vi "interp type 2.vi"(1 "NaN":dbl[][](array[numeric]) format="%.2f", 2 "Remove front and end":bool) -> (0 "Interpolated":dbl[][](array[numeric]) format="%.2f")   [LabVIEW 2016]
uses:
  <vilib>/Analysis/1siggen.llb/Ramp Pattern by Samples.vi
  <vilib>/Analysis/NI_AALBase.lvlib
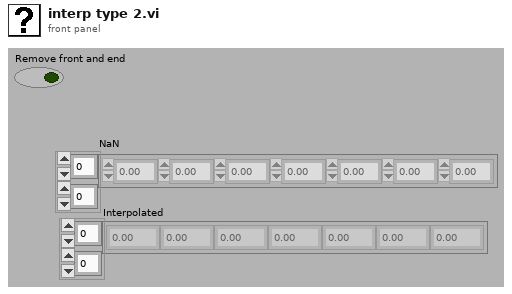
[diagram p1: front panel]
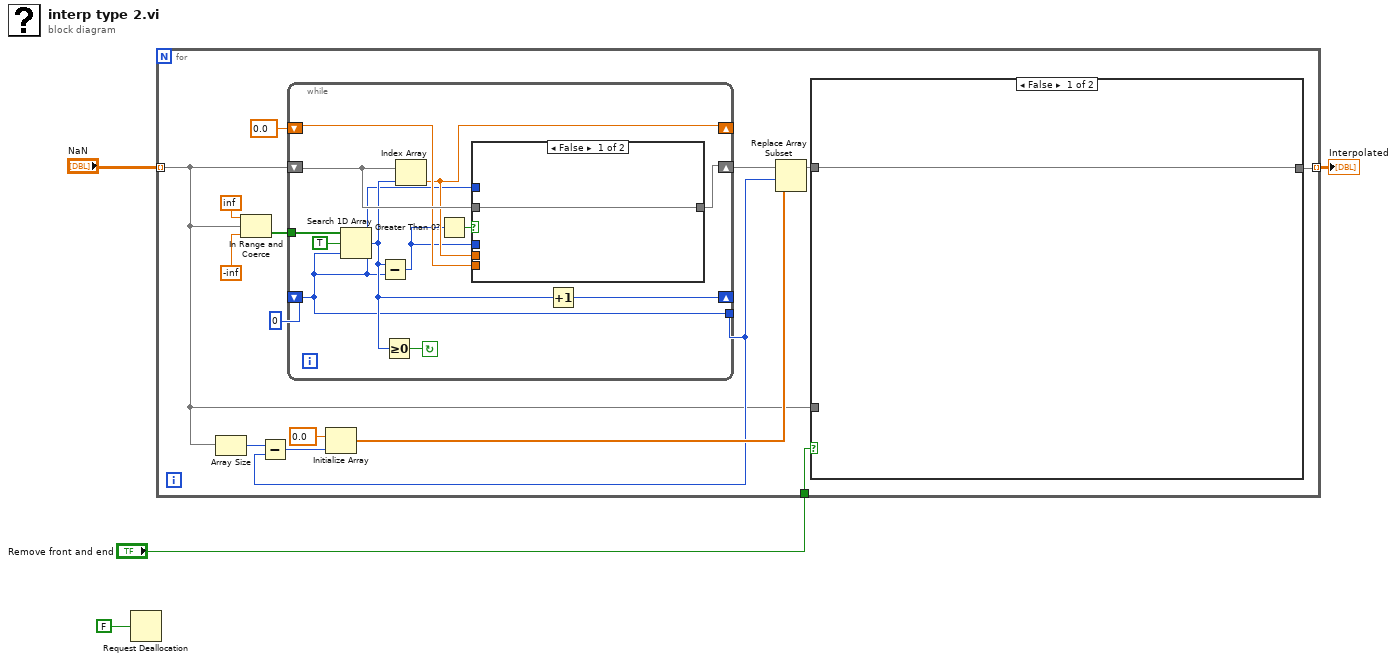
[diagram p0: block diagram]
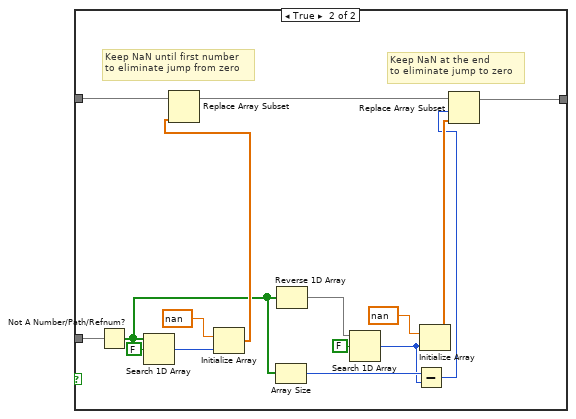
[diagram p2: hidden frame]
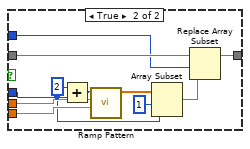
[diagram p3: hidden frame]
diagram:
  n1 = Request Deallocation(FALSE ("flag")) -> ()
  n2 = for {
    tunnel: "NaN" -> [w8] mode=indexing
    tunnel: [w6] -> w3 mode=indexing
    tunnel: "Remove front and end" -> [w5]
    n3 = Array Size(array=w8) -> (size(s)=w14:i32)
    n4 = In Range and Coerce(upper limit=inf, x=w8, lower limit=-inf) -> (In Range?=w17:bool[])  [unwired: 1 out]
    n5 = while {
      tunnel: w17 -> [w48]
      shift-right: [w38] -> _
      shift-left: 0 -> [w37]
      shift-right: [w43] -> w11
      shift-left: w8 -> [w46]
      shift-right: [w44] -> _
      shift-left: 0.0 ("Numeric") -> [w45]
      tunnel: [w37] -> w9
      stop <- w41 continue-if-true
      n6 = Search 1D Array(1D array=w48, element=TRUE, start index (0)=w37) -> (index of element=w42:i32)
      n7 = Subtract(x=w42, y=w37) -> (x-y=w39:i32)
      n8 = Greater Or Equal To 0?(x=w42) -> (x >= 0?=w41:bool)
      n9 = Index Array(array=w46, index=w42) -> (element=w44:dbl)
      n10 = Greater Than 0?(x=w39) -> (x > 0?=w40:bool)
      n11 = case shown="False" w40 {
        tunnel: w46 -> [w49 w60]
        tunnel: w45 -> [_ w59]
        tunnel: w44 -> [_ w58]
        tunnel: [w49 w57] -> w43
        tunnel: w39 -> [_ w52]
        tunnel: w37 -> [_ w50]
        frame False {
        }
        frame True {
          n12 = Add(x=2, y=w52) -> (x+y=w56:i32)
          n13 = call-poly <vilib>:"Ramp Pattern.vi"("start"=w59, "end"=w58, "samples"=w56) -> ("Ramp Pattern"=w54:dbl[])  [unwired: 7 in, 1 out]
          n14 = Array Subset(array=w54, index=1, length=w52) -> (w51:dbl[])
          n15 = Replace Array Subset(array=w60, new element=w51, index=w50) -> (w57:dbl[])
        }
      }
      n16 = Increment(x=w42) -> (x+1=w38:i32)
    }
    n17 = Subtract(x=w14, y=w9) -> (x-y=w13:i32)
    n18 = Initialize Array(0.0 ("element"), w13) -> (w10:dbl[])
    n19 = Replace Array Subset(array=w11, new element=w10, index=w9) -> (w7:dbl[])
    n20 = case shown="False" w5 {
      tunnel: w8 -> [_ w36]
      tunnel: w7 -> [w20 w35]
      tunnel: [w20 w34] -> w6
      frame False {
      }
      frame True {
        # "Keep NaN at the end \nto eliminate jump to zero"
        # "Keep NaN until first number\nto eliminate jump from zero"
        n21 = Not A Number/Path/Refnum?(number/path/refnum=w36) -> (NaN/Path/Refnum?=w26:bool[])
        n22 = Search 1D Array(1D array=w26, element=FALSE) -> (index of element=w22:i32)  [unwired: 1 in]
        n23 = Initialize Array(nan ("element"), w22) -> (w31:dbl[])
        n24 = Replace Array Subset(array=w35, new element=w31) -> (w27:dbl[])  [unwired: 1 in]
        n25 = Array Size(array=w26) -> (size(s)=w25:i32)
        n26 = Reverse 1D Array(array=w26) -> (reversed array=w28:bool[])
        n27 = Search 1D Array(1D array=w28, element=FALSE) -> (index of element=w21:i32)  [unwired: 1 in]
        n28 = Subtract(x=w25, y=w21) -> (x-y=w23:i32)
        n29 = Initialize Array(nan ("element"), w21) -> (w24:dbl[])
        n30 = Replace Array Subset(array=w27, new element=w24, index=w23) -> (w34:dbl[])
      }
    }
  }
  "Interpolated" <- w3
